vi "Trigger Detection for 1 Channel (obs).vi"(0 "signal in":waveform(dbl), 1 "reset":bool, 5 "level":dbl format="%.2p", 7 "hysteresis":dbl format="%.2p", 9 "location mode":u16(ring) items=["Index", "Time"], 11 "error in (no error)":errorcluster, 12 "trigger slope":u16(ring)=1 items=["Falling Edge", "Rising Edge"]) -> (4 "trigger location":dbl format="%0.2f", 8 "trigger detected?":bool, 15 "error out":errorcluster)   [LabVIEW 2020, in "NI_MAPro.lvlib"]
doc: "Finds the first level-crossing location in a waveform. You can retrieve the trigger location as an index or as a time. The trigger conditions are specified in terms of threshold <B>level</B>, <B>slope</B>, and <B>hysteresis</B>. The data type you wire to the <B>signal in</B> input determines the polymorphic instance to use."
uses:
  NI_MAPro.lvlib
  NI_MABase.lvlib
  <resource>/lvanlys.dll
panel:
  out "number of triggers detected":i32
  in  "max number trigger pts":i32=1
  # "This VI is obsolete !!!\n\nNOTE: This obsolete VI uses the ending value in last data block as the instruction for the initial status of current data block. The new Trigger Detection VI uses the ending status instead."
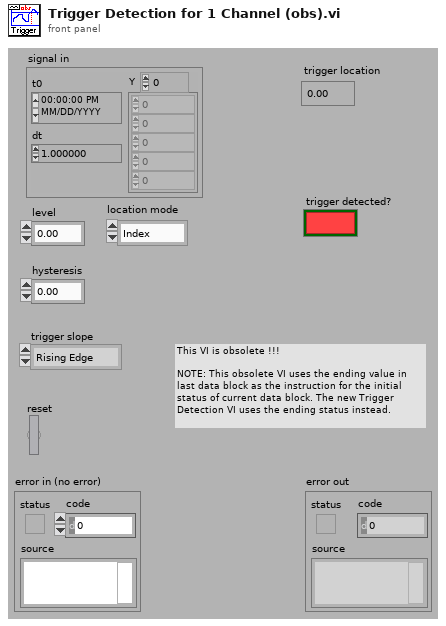
[diagram p1: front panel]
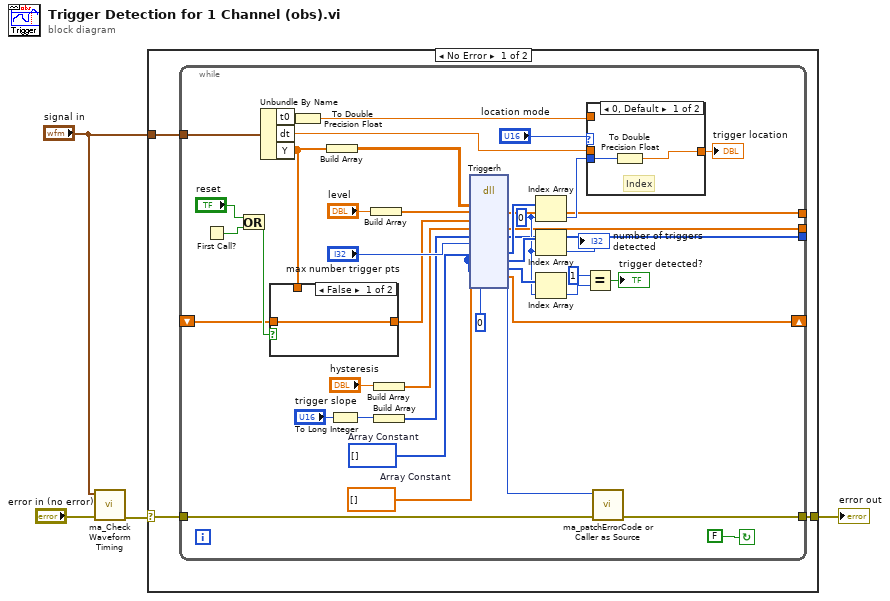
[diagram p0: block diagram]
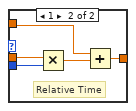
[diagram p2: hidden frame]
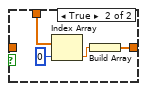
[diagram p3: hidden frame]
diagram:
  n1 = call "ma_Check Waveform Timing.vi"("error in (no error)"="error in (no error)", "signal in"="signal in") -> ("error out"=w2:errorcluster)  [unwired: 1 in, 8 out]
  n2 = case shown="No Error" w2 {
    selector: w2 -> [w7 w61]
    tunnel: [w6 w61] -> w4
    tunnel: "signal in" -> [w5 _]
    frame No Error {
      n3 = while {
        tunnel: w7 -> [w13]
        tunnel: [w12] -> w6
        shift-right: [w37] -> _
        shift-left: _ -> [w33]
        tunnel: w5 -> [w14]
        tunnel: [w10] -> _
        tunnel: [w9] -> _
        tunnel: [w8] -> _
        stop <- FALSE continue-if-true
        w38 = 0 ("Index")
        w45 = dbl[] []  # Array Constant
        w15 = i32[] []  # Array Constant
        n4 = First Call?() -> (First Call?: T/F=w17:bool)
        n5 = Or(x="reset", y=w17) -> (x .or. y?=w35:bool)
        n6 = Unbundle By Name(w14) -> ("t0"=w18:timestamp, "dt"=w20:dbl, "Y"=w34:dbl[])
        n7 = case shown="False" w35 {
          tunnel: w34 -> [_ w60]
          tunnel: [w56 w58] -> w32
          tunnel: w33 -> [w56 _]
          frame False {
          }
          frame True {
            n8 = Index Array(array=w60, index=0 ("Index")) -> (element=w57:dbl)
            n9 = Build Array(w57) -> (w58:dbl[])
          }
        }
        n10 = To Double Precision Float(number=w18) -> (double precision float=w19:dbl)
        n11 = Build Array(w34) -> (w24:dbl[][])
        n12 = To Long Integer(number="trigger slope") -> (32bit integer=w26:i32)
        n13 = Build Array("level") -> (w30:dbl[])
        n14 = Build Array("hysteresis") -> (w28:dbl[])
        n15 = Build Array(w26) -> (w25:i32[])
        n16 = dll-call lib="C:/Program Files (x86)/National Instruments/LabVIEW 2020/resource/lvanlys.*" fn="Triggerh"("x"=w24, "level"=w30, "initial"=w32, "hysterisis"=w28, "slope"=w25, "nptsH"="max number trigger pts", "triggerIndex"=w15, "number_of_triggers_detected"=w15, "triggerDetectedbyte"=w15, "final"=w45, "error"=0) -> ("level"=w10:dbl[], "hysterisis"=w9:dbl[], "slope"=w8:i32[], "triggerIndex"=w44:i32[], "number_of_triggers_detected"=w43:i32[], "triggerDetectedbyte"=w41:i32[], "final"=w37:dbl[], "error"=w11:i32)  [unwired: 6 in, 3 out]
        n17 = Index Array(array=w44, index=w38) -> (element=w23:i32)
        n18 = Index Array(array=w43, index=w38) -> (element=→"number of triggers detected":i32)
        n19 = Index Array(array=w41, index=w38) -> (element=w40:i32)
        n20 = Equal?(x=1 ("Element Data"), y=w40) -> (x = y?=→"trigger detected?":bool)
        n21 = case shown="0, Default" "location mode" {
          tunnel: w23 -> [w50 w55]
          tunnel: [w49 w51] -> w21
          tunnel: w20 -> [_ w54]
          tunnel: w19 -> [_ w52]
          frame 0, Default {
            # "Index"
            n22 = To Double Precision Float(number=w50) -> (double precision float=w49:dbl)
          }
          frame 1 {
            # "Relative Time"
            n23 = Multiply(x=w54, y=w55) -> (x*y=w53:dbl)
            n24 = Add(x=w52, y=w53) -> (x+y=w51:dbl)
          }
        }
        "trigger location" <- w21
        n25 = call "ma_patchErrorCode or Caller as Source.vi"("error in (no error)"=w13, "error code"=w11) -> ("error out"=w12:errorcluster)  [unwired: 2 in, 7 out]
      }
    }
    frame Error {
    }
  }
  "error out" <- w4
